vi "AFT Create FIR Normalized Filtered-X LMS.vi"(7 "secondary path":dbl[](array[numeric]), 8 "error in (no error)":errorcluster, 10 "step size":dbl=0.01, 11 "filter length":i32=128) -> (0 "error out":errorcluster, 3 "filtered-x adaptive filter out":refnum<k20>)   [LabVIEW 2017, in "NI_AdaptiveFilter.lvlib"]
doc: "Creates a finite impulse response (FIR) adaptive filter with the normalized filtered-x least mean squares (LMS) algorithm."
uses:
  <vilib>/addons/Adaptive Filters/NI_AdaptiveFilter.lvlib
  <resource>/AdaptiveFilters.dll
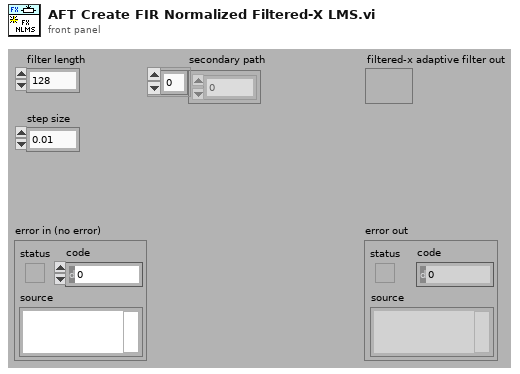
[diagram p1: front panel]
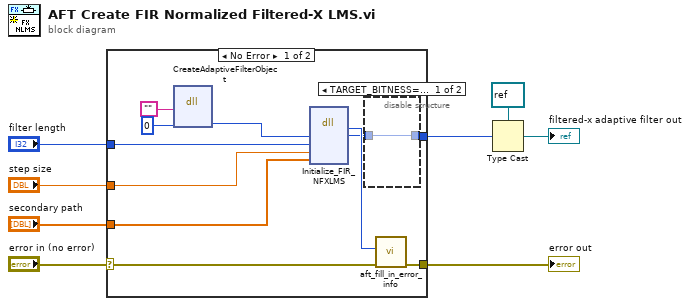
[diagram p0: block diagram]
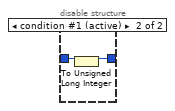
[diagram p2: hidden frame]
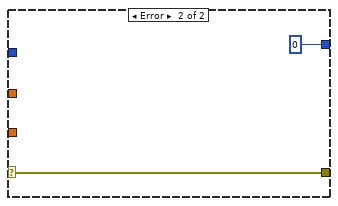
[diagram p3: hidden frame]
diagram:
  n1 = case shown="No Error" "error in (no error)" {
    selector: "error in (no error)" -> [w13 w24]
    tunnel: [w12 w24] -> w7
    tunnel: "filter length" -> [w16 _]
    tunnel: "step size" -> [w15 _]
    tunnel: [w10 u32 0 ("pSession")] -> w3
    tunnel: "secondary path" -> [w11 _]
    frame No Error {
      n2 = dll-call lib="C:/Program Files/National Instruments/LabVIEW 2017/resource/AdaptiveFilters.*" fn="CreateAdaptiveFilterObject" ("Complex Data Create")("UnusedReferenceName"="", "pConfigurationHandle"=u32 0 ("pScriptRefNum")) -> ("pConfigurationHandle"=w17:u64)  [unwired: 3 in, 4 out]
      n3 = dll-call lib="C:/Program Files/National Instruments/LabVIEW 2017/resource/AdaptiveFilters.*" fn="Initialize_FIR_NFXLMS" ("Complex Data Initialization")("pSession"=w17, "order"=w16, "mu"=w15, "SecondaryPath"=w11) -> ("err"=w14:i32, "pSession"=w9:u64)  [unwired: 6 in, 2 out]
      n4 = disable-structure shown="TARGET_BITNESS==64, Default" {
        disable-tunnel: w9 -> [w20 w22]
        disable-tunnel: [w20 w21] -> w10
        frame condition #0 {
        }
        frame condition #1 (active) {
          n5 = To Unsigned Long Integer(number=w22) -> (unsigned 32bit integer=w21:u32)
        }
      }
      n6 = call <vilib>:"aft_fill_in_error_info.vi"("error in"=w13, "status code"=w14) -> ("error out"=w12:errorcluster)  [unwired: 2 in, 7 out]
    }
    frame Error {
    }
  }
  "error out" <- w7
  n7 = Type Cast(type=refnum<k20> refnum ("reference"), x=w3) -> (*(type *) &x=→"filtered-x adaptive filter out":refnum<k20>)
